vi "poly_is_running_state.vi"(4 "execution state":T1(ring)) -> (1 "running top level?":bool)   [LabVIEW 2015, in "_ref_tools_polys.lvlib"]
uses:
  _ref_tools_polys.lvlib
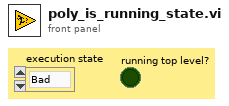
[diagram p1: front panel]
types:
  T1 = enum32{"Bad", "Idle", "Run top level", "Running"}
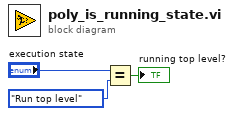
[diagram p0: block diagram]
diagram:
  n1 = Equal?(x="execution state", y=T1."Run top level") -> (x = y?=→"running top level?":bool)
